vi "Calculate Built Version.vi"(0 "NIPKG_LV in":refnum<class "NIPKG_LV.lvclass">, 11 "error in (no error)":errorcluster) -> (4 "NIPKG_LV out":refnum<class "NIPKG_LV.lvclass">, 15 "error out":errorcluster)   [LabVIEW 2017, in "CL_G3_VIComponentBuilder.lvlib" / "NIPKG_LV.lvclass"]
uses:
  NIPKG_LV.lvclass
  C:/builds/Component BuilderBT/SrcDist/Exports/Exports/Export.lvclass
  C:/builds/Component BuilderBT/SrcDist/Exports/NI Build Specification_LV/NI Build Specification_LV.lvclass
  Exports/Export.lvclass/Export.ctl
  NI Build Specification_LV/NI Build Specification_LV.lvclass/NI Build Specification_LV.ctl
  Exports/Accessors/Read Exported Build Specification Path.vi
  NI Build Specification_LV/Accessors/Read Build Number XML Prop Name.vi
  Exports/Accessors/Write Built Version.vi
  <vilib>/xml/Load XML File.vi
  <vilib>/xml/Close Reference(Node).vi
  <vilib>/xml/NI_XML.lvlib
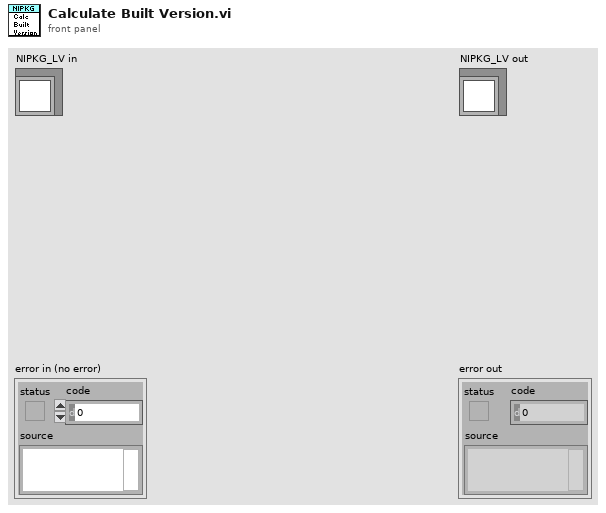
[diagram p1: front panel]
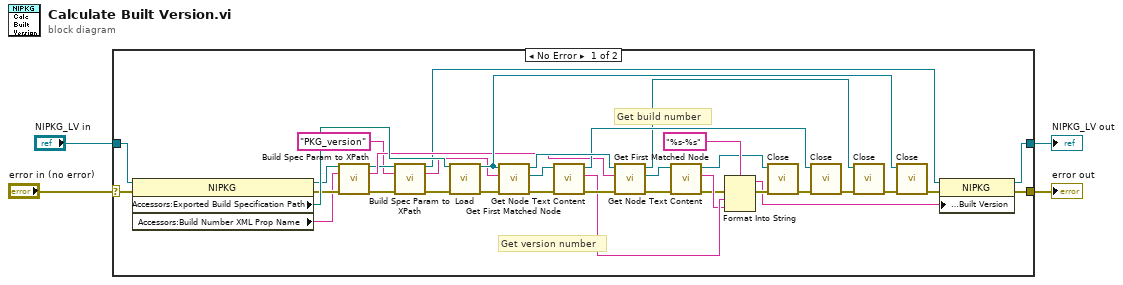
[diagram p0: block diagram]
diagram:
  n1 = case shown="No Error" "error in (no error)" {
    selector: "error in (no error)" -> [w39 w41]
    tunnel: "NIPKG_LV in" -> [w40 w42]
    tunnel: [w38 w42] -> w4
    tunnel: [w25 w41] -> w3
    frame No Error {
      # "Get build number"
      # "Get version number"
      n2 = property class="NIPKG"(reference=w40, error in=w39) -> (reference out=w14:refnum<class "NIPKG_LV.lvclass">, error out=w12:errorcluster, "Accessors:Exported Build Specification Path"=w34:path, "Accessors:Build Number XML Prop Name"=w9:string)
      n3 = call-dynamic "Build Spec Param to XPath.vi"("NI Build Specification"=w14, "Build Spec Parameter Name"=w9, "error in (no error)"=w12) -> ("NI Build Specification"=w11:refnum<class "NIPKG_LV.lvclass">, "XPath to the specific build Spec Property"=w13:string, "error out"=w8:errorcluster)  [unwired: 10 in]
      n4 = call-dynamic "Build Spec Param to XPath.vi"("NI Build Specification"=w11, "Build Spec Parameter Name"="PKG_version", "error in (no error)"=w8) -> ("NI Build Specification"=w6:refnum<class "NIPKG_LV.lvclass">, "XPath to the specific build Spec Property"=w10:string, "error out"=w7:errorcluster)  [unwired: 10 in]
      n5 = call-poly <vilib>:"Load.vi"("path to XML document"=w34, "error in (no error)"=w7) -> ("DOM document out"=w17:refnum<k20>, "error out"=w35:errorcluster)  [unwired: 11 in, 1 out]
      n6 = call <vilib>:"Get First Matched Node.vi"("error in (no error)"=w35, "XPath expression"=w10, "node in"=w17) -> ("error out"=w36:errorcluster, "node result"=w37:refnum<k20>, "node out"=w32:refnum<k20>)  [unwired: 6 in]
      n7 = call <vilib>:"Get Node Text Content.vi"("error in (no error)"=w36, "node in"=w37) -> ("error out"=w33:errorcluster, "node text"=w28:string, "node out"=w21:refnum<k20>)  [unwired: 7 in]
      n8 = call <vilib>:"Get First Matched Node.vi"("error in (no error)"=w33, "XPath expression"=w13, "node in"=w32) -> ("error out"=w30:errorcluster, "node result"=w31:refnum<k20>, "node out"=w20:refnum<k20>)  [unwired: 6 in]
      n9 = call <vilib>:"Get Node Text Content.vi"("error in (no error)"=w30, "node in"=w31) -> ("error out"=w26:errorcluster, "node text"=w27:string, "node out"=w23:refnum<k20>)  [unwired: 7 in]
      n10 = Format Into String(format string="%s-%s", error in=w26, w28, w27) -> (resulting string=w15:string, error out=w24:errorcluster)  [unwired: 1 in]
      n11 = call-poly <vilib>:"Close.vi"("error in (no error)"=w24, "node"=w23) -> ("error out"=w22:errorcluster)  [unwired: 7 in]
      n12 = call-poly <vilib>:"Close.vi"("error in (no error)"=w22, "node"=w21) -> ("error out"=w19:errorcluster)  [unwired: 7 in]
      n13 = call-poly <vilib>:"Close.vi"("error in (no error)"=w19, "node"=w20) -> ("error out"=w18:errorcluster)  [unwired: 7 in]
      n14 = call-poly <vilib>:"Close.vi"("error in (no error)"=w18, "node"=w17) -> ("error out"=w16:errorcluster)  [unwired: 7 in]
      n15 = property class="NIPKG"(reference=w6, error in=w16, "Accessors:Built Version"=w15) -> (reference out=w38:refnum<class "NIPKG_LV.lvclass">, error out=w25:errorcluster)
    }
    frame Error {
    }
  }
  "error out" <- w3
  "NIPKG_LV out" <- w4
